vi "Add Entries.vi"(7 "Flat View?":bool, 8 "error in":errorcluster, 10 "VI Data":T1[](array[typedef]), 11 "Tree Map in":refnum<class "Project Tree Map.lvclass">) -> (0 "error out":errorcluster, 3 "Tree Map out":refnum<class "Project Tree Map.lvclass">)   [LabVIEW 2020, in "Project Tree.lvlib" / "Project Tree Map.lvclass"]
uses:
  Project Tree Map.lvclass
  <vilib>/picture/picture.llb/imagedata.ctl
  CTLs/VI Properties.ctl
  VI Properties Editor.lvlib
  CTLs/Control Properties.ctl
  CTLs/VI Data.ctl
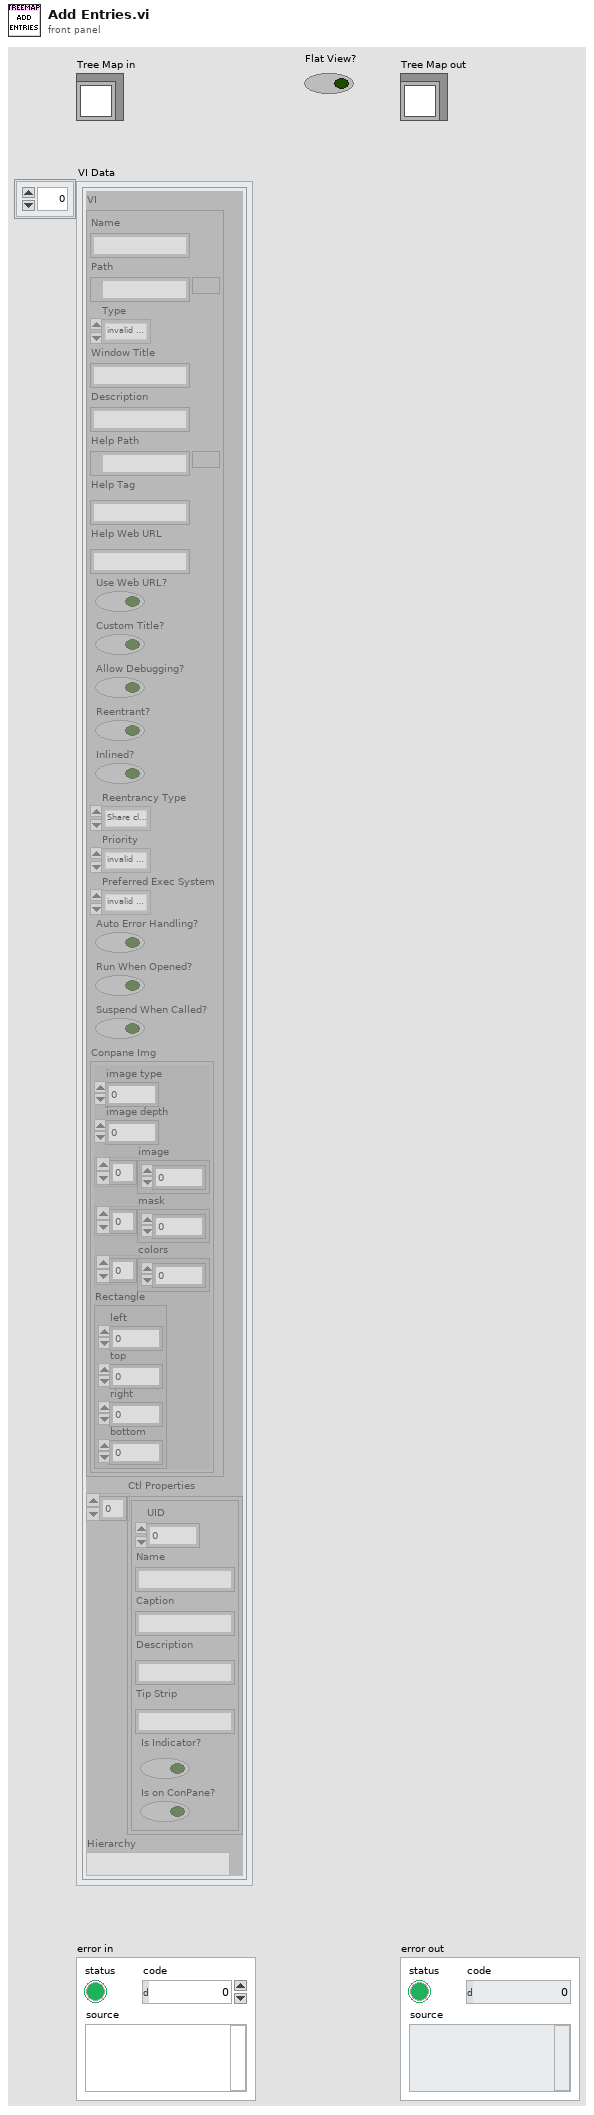
[diagram p1: front panel]
types:
  T1 = typedef "VI Properties Editor.lvlib/VI Data.ctl" = cluster{"VI":T2, "Ctl Properties":T4[], "Hierarchy":string}
  T2 = typedef "VI Properties Editor.lvlib/VI Properties.ctl" = cluster{"Name":string, "Path":path, "Type":enum32{"invalid VI type", "Standard VI", "Control VI", "Global VI", "Polymorphic VI", "Configuration VI", "SubSystem", "Facade VI", "Method VI", "Statechart Diagram VI"}, "Window Title":string, "Description":string, "Help Path":path, "Help Tag":string, "Help Web URL":string, "Use Web URL?":bool, "Custom Title?":bool, "Allow Debugging?":bool, "Reentrant?":bool, "Inlined?":bool, "Reentrancy Type":enum16{"Share clones between instances", "Preallocate clone for each instance"}, "Priority":enum32{"invalid priority", "background priority", "normal priority", "above normal priority", "high priority", "time critical priority", "subroutine"}, "Preferred Exec System":enum32{"invalid execution system", "user interface", "standard", "instrument i/o", "data acquisition", "other 1", "other 2", "same as caller"}, "Auto Error Handling?":bool, "Run When Opened?":bool, "Suspend When Called?":bool, "Conpane Img":T3}
  T3 = typedef "imagedata.ctl" = cluster{"image type":i32, "image depth":i32, "image":u8[], "mask":u8[], "colors":u32[], "Rectangle":cluster{"left":i16, "top":i16, "right":i16, "bottom":i16}}
  T4 = typedef "VI Properties Editor.lvlib/Control Properties.ctl" = cluster{"UID":i32, "Name":string, "Caption":string, "Description":string, "Tip Strip":string, "Is Indicator?":bool, "Is on ConPane?":bool}
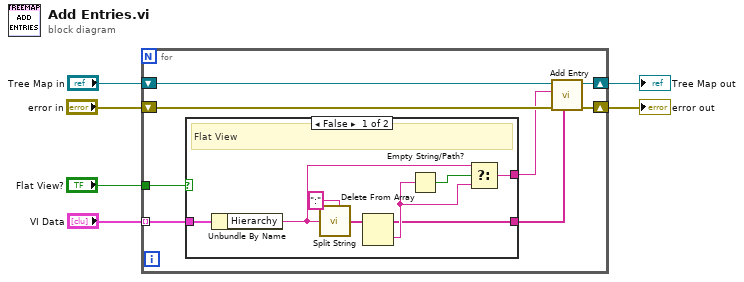
[diagram p0: block diagram]
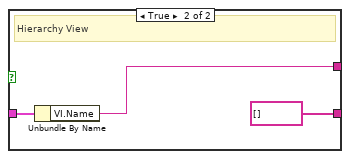
[diagram p2: hidden frame]
diagram:
  n1 = for {
    tunnel: "VI Data" -> [w13] mode=indexing
    shift-right: [w11] -> w3
    shift-left: "Tree Map in" -> [w14]
    shift-right: [w10] -> w2
    shift-left: "error in" -> [w12]
    tunnel: "Flat View?" -> [w7]
    n2 = case shown="False" w7 {
      tunnel: w13 -> [w22 w25]
      tunnel: [w16 string[] [] ("Split String")] -> w9
      tunnel: [w15 w24] -> w8
      frame False {
        # "Flat View"
        n3 = Unbundle By Name(w22) -> ("Hierarchy"=w20:string)
        n4 = call <vilib>:"Split String.vi"("Split Pattern"=":", "Input String"=w20) -> ("Split String"=w19:string[])  [unwired: 5 in]
        n5 = Delete From Array(array=w19) -> (deleted portion=w17:string, array with subset deleted=w16:string[])  [unwired: 2 in]
        n6 = Empty String/Path?(string/path=w17) -> (empty?=w18:bool)
        n7 = Select(t=w20, s=w18, f=w17) -> (s? t:f=w15:string)
      }
      frame True {
        # "Hierarchy View"
        n8 = Unbundle By Name(w25) -> ("VI.Name"=w24:string)
      }
    }
    n9 = call "Add Entry.vi"("Parent (None)"=w9, "error in"=w12, "Name"=w8, "Tree Map in"=w14) -> ("error out"=w10:errorcluster, "Tree Map out"=w11:refnum<class "Project Tree Map.lvclass">)  [unwired: 5 in, 1 out]
  }
  "Tree Map out" <- w3
  "error out" <- w2
